vi "Motor_stagedelay.vi"(0 "Acceleration":dbl format="%#_8g", 1 "MAX Speed":dbl, 2 "Min X":dbl=1.0 min=0.0, 3 "Max X":dbl=1.0 min=0.0, 4 "Step size Y":dbl=1.0 min=0.0, 5 "Step size X":dbl=1.0 min=0.0) -> (14 "Travel time short (ms)":dbl, 19 "Travel time long (ms)":dbl)   [LabVIEW 2016]
panel:
  out "Distance long":dbl
  out "Acceleration distance":dbl
  out "Acceleration time":dbl
  out "Distance_short":dbl
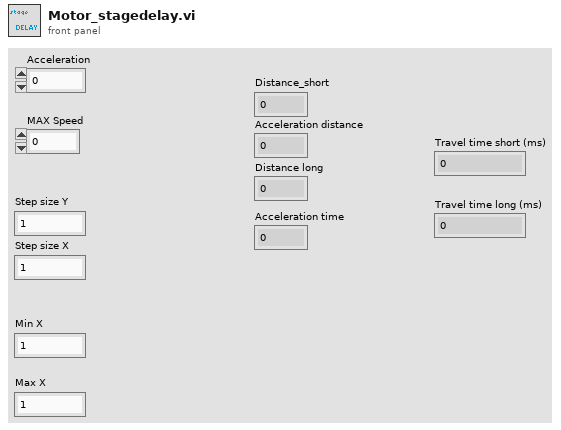
[diagram p1: front panel]
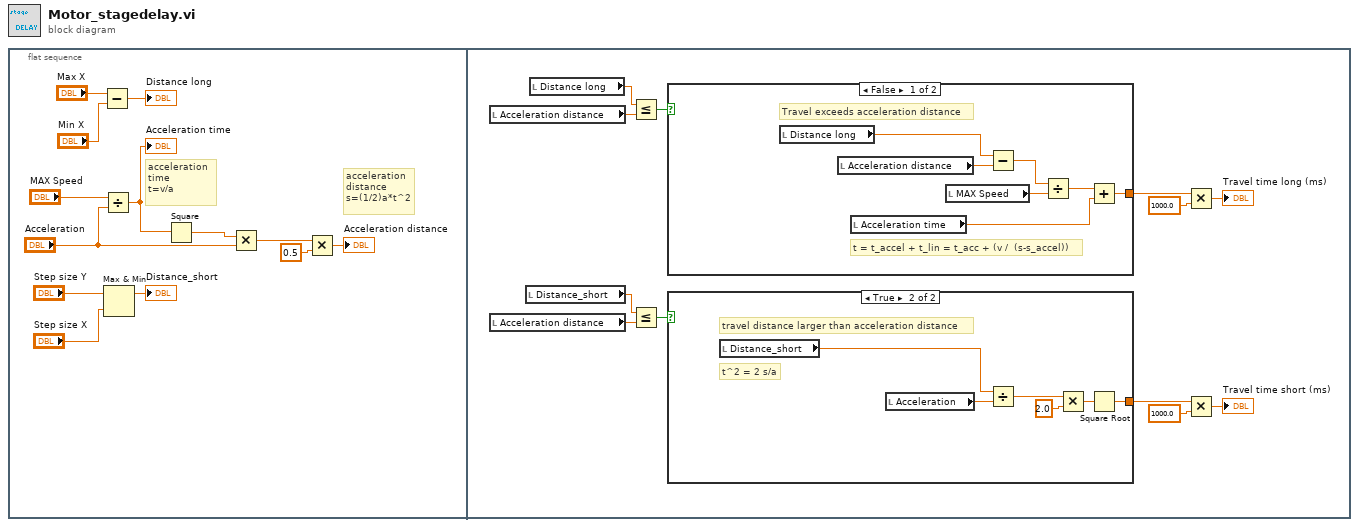
[diagram p0: block diagram]
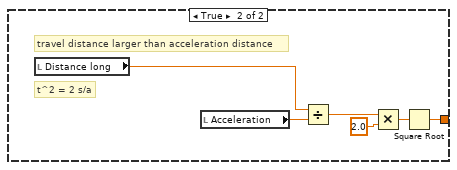
[diagram p2: hidden frame]
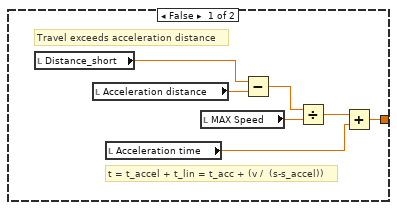
[diagram p3: hidden frame]
diagram:
  n1 = flat-sequence {
    frame #0 {
      # "acceleration \ndistance\ns=(1/2)a*t^2"
      # "acceleration \ntime\nt=v/a"
      n2 = Subtract(x="Max X", y="Min X") -> (x-y=→"Distance long":dbl)
      n3 = Divide(x="MAX Speed", y="Acceleration") -> (x/y=w9:dbl)
      "Acceleration time" <- w9
      n4 = Max & Min(x="Step size Y", y="Step size X") -> (max(x,y)=→"Distance_short":dbl)  [unwired: 1 out]
      n5 = Square(x=w9) -> (x^2=w8:dbl)
      n6 = Multiply(x=w8, y="Acceleration") -> (x*y=w6:dbl)
      n7 = Multiply(x=w6, y=0.5) -> (x*y=→"Acceleration distance":dbl)
    }
    frame #1 {
      n8 = local read "Acceleration distance"() -> (w22:dbl)
      n9 = local read "Acceleration distance"() -> (w25:dbl)
      n10 = local read "Distance_short"() -> (w24:dbl)
      n11 = local read "Distance long"() -> (w21:dbl)
      n12 = Less Or Equal?(x=w21, y=w22) -> (x <= y?=w20:bool)
      n13 = Less Or Equal?(x=w24, y=w25) -> (x <= y?=w23:bool)
      n14 = case shown="False" w20 {
        tunnel: [w30 w33] -> w14
        frame False {
          # "t = t_accel + t_lin = t_acc + (v /  (s-s_accel))"
          # "Travel exceeds acceleration distance"
          n15 = local read "Distance long"() -> (w32:dbl)
          n16 = local read "Acceleration distance"() -> (w31:dbl)
          n17 = local read "Acceleration time"() -> (w28:dbl)
          n18 = local read "MAX Speed"() -> (w27:dbl)
          n19 = Subtract(x=w32, y=w31) -> (x-y=w26:dbl)
          n20 = Divide(x=w26, y=w27) -> (x/y=w29:dbl)
          n21 = Add(x=w29, y=w28) -> (x+y=w30:dbl)
        }
        frame True {
          # "t^2 = 2 s/a"
          # "travel distance larger than acceleration distance"
          n22 = local read "Distance long"() -> (w35:dbl)
          n23 = local read "Acceleration"() -> (w36:dbl)
          n24 = Divide(x=w35, y=w36) -> (x/y=w37:dbl)
          n25 = Multiply(x=w37, y=2.0) -> (x*y=w34:dbl)
          n26 = Square Root(x=w34) -> (sqrt(x)=w33:dbl)
        }
      }
      n27 = case shown="True" w23 {
        tunnel: [w43 w46] -> w17
        frame False {
          # "t = t_accel + t_lin = t_acc + (v /  (s-s_accel))"
          # "Travel exceeds acceleration distance"
          n28 = local read "Distance_short"() -> (w45:dbl)
          n29 = local read "Acceleration distance"() -> (w44:dbl)
          n30 = local read "Acceleration time"() -> (w41:dbl)
          n31 = local read "MAX Speed"() -> (w40:dbl)
          n32 = Subtract(x=w45, y=w44) -> (x-y=w39:dbl)
          n33 = Divide(x=w39, y=w40) -> (x/y=w42:dbl)
          n34 = Add(x=w42, y=w41) -> (x+y=w43:dbl)
        }
        frame True {
          # "t^2 = 2 s/a"
          # "travel distance larger than acceleration distance"
          n35 = local read "Distance_short"() -> (w48:dbl)
          n36 = local read "Acceleration"() -> (w49:dbl)
          n37 = Divide(x=w48, y=w49) -> (x/y=w50:dbl)
          n38 = Multiply(x=w50, y=2.0) -> (x*y=w47:dbl)
          n39 = Square Root(x=w47) -> (sqrt(x)=w46:dbl)
        }
      }
      n40 = Multiply(x=w14, y=1000.0) -> (x*y=→"Travel time long (ms)":dbl)
      n41 = Multiply(x=w17, y=1000.0) -> (x*y=→"Travel time short (ms)":dbl)
    }
  }
